vi "Error Cluster From Win32 Error Code.vi"(7 "is warning? (False)":bool, 8 "error in (no error)":errorcluster, 10 "additional message (\"\")":string, 11 "error code (0)":i32) -> (0 "error out":errorcluster)   [LabVIEW 2020]
doc: "Converts an error or warning code to an error cluster. This VI is useful when you receive a return value from a DLL call or when you return user-defined error codes."
uses:
  kernel32.dll
panel:
  in  "buffer size (65535)":u32=65535
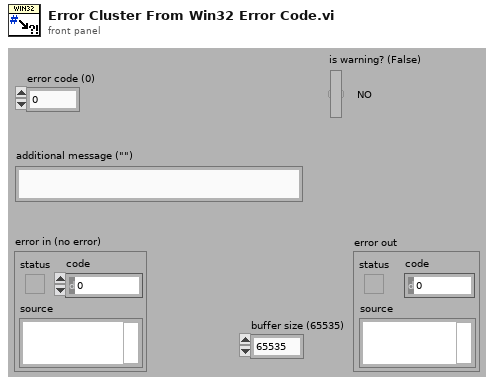
[diagram p1: front panel]
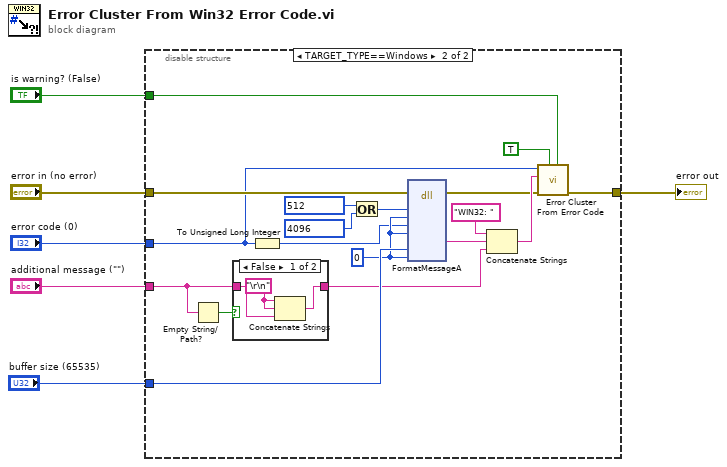
[diagram p0: block diagram]
diagram:
  n1 = disable-structure shown="TARGET_TYPE==Windows" {
    disable-tunnel: [w7 w25] -> w6
    disable-tunnel: "error in (no error)" -> [w7 w24]
    disable-tunnel: "error code (0)" -> [_ w23]
    disable-tunnel: "additional message (\"\")" -> [_ w8]
    disable-tunnel: "is warning? (False)" -> [_ w20]
    disable-tunnel: "buffer size (65535)" -> [_ w19]
    frame condition #0 {
    }
    frame condition #1 (active) {
      w15 = u32 0 ("nSize")
      n2 = Empty String/Path?(string/path=w8) -> (empty?=w10:bool)
      n3 = case shown="False" w10 {
        tunnel: [w27 w29] -> w9
        tunnel: w8 -> [w28 w29]
        frame False {
          w26 = "\r\n"
          n4 = Concatenate Strings(w26, w26, w28) -> (w27:string)
        }
        frame True {
        }
      }
      n5 = To Unsigned Long Integer(number=w23) -> (unsigned 32bit integer=w12:u32)
      n6 = Or(x=u32 512, y=u32 4096) -> (x .or. y?=w16:u32)
      n7 = dll-call lib="kernel32.dll" fn="FormatMessageA"(error in=w24, "dwFlags"=w16, "lpSource"=w15, "dwMessageId"=w12, "dwLanguageId"=w15, "nSize"=w19, "Arguments"=w15) -> (error out=w21:errorcluster, "lpBuffer"=w14:string)  [unwired: 6 in, 5 out]
      n8 = Concatenate Strings("WIN32: " ("string"), w14, w9) -> (w22:string)
      n9 = call <vilib>:"Error Cluster From Error Code.vi"("is warning? (False)"=w20, "show call chain? (False)"=TRUE, "error in (no error)"=w21, "error message (\"\")"=w22, "error code (0)"=w23) -> ("error out"=w25:errorcluster)  [unwired: 4 out]
    }
  }
  "error out" <- w6
